vi "Get Tunnel Position on Structure.vi"(8 "error in":errorcluster, 11 "Tunnel Ref":refnum<vi>) -> (0 "error out":errorcluster, 1 "Class Name":string, 2 "Position":cluster{"Left":i32, "Top":i32}, 3 "Tunnel Position":enum16{"Left", "Top", "Right", "Bottom"}(ring))   [LabVIEW 2023]
uses:
  <userlib>/_OpenG.lib/array/array.llb/openg_array.lvlib
panel:
  out "Structure Bounds":T1
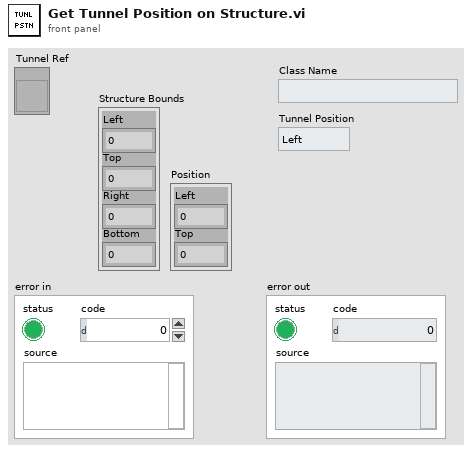
[diagram p1: front panel]
types:
  T1 = cluster{"Left":i16, "Top":i16, "Right":i16, "Bottom":i16}
  T2 = typedef "LVRectTypeDef.ctl" = cluster{"Left":i16, "Top":i16, "Right":i16, "Bottom":i16}
  T3 = typedef "LVPositionTypeDef.ctl" = cluster{"Left":i32, "Top":i32}
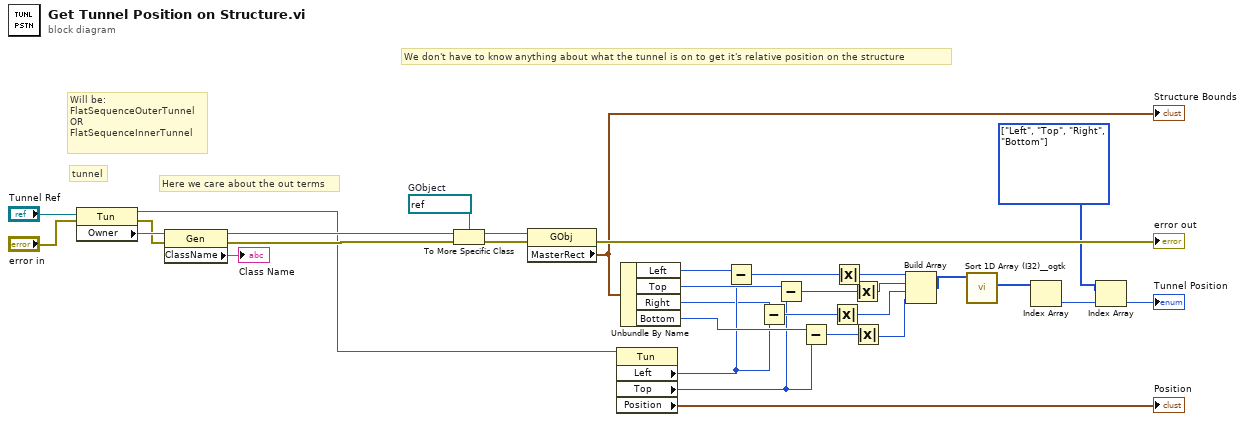
[diagram p0: block diagram]
diagram:
  w19 = enum16{"Left", "Top", "Right", "Bottom"}[] [enum."Left", enum."Top", enum."Right", enum."Bottom"] items=["Left", "Top", "Right", "Bottom"]
  w2 = refnum<vi> refnum  # GObject
  # "We don't have to know anything about what the tunnel is on to get it's relative position on the structure"
  # "Here we care about the out terms"
  # "Will be:\nFlatSequenceOuterTunnel\nOR\nFlatSequenceInnerTunnel"
  # "tunnel"
  n1 = property class="Tun"(reference="Tunnel Ref", error in="error in") -> (reference out=w23:refnum<vi>, error out=w28:errorcluster, "Owner"=w31:refnum<vi>)
  n2 = property class="Gen"(reference=w31, error in=w28) -> (error out=w27:errorcluster, "ClassName"=→"Class Name":string)  [unwired: 1 out]
  n3 = To More Specific Class(target class=w2, reference=w31, error in=w27) -> (specific class reference=w3:refnum<vi>, error out=w1:errorcluster)
  n4 = property class="GObj"(reference=w3, error in=w1) -> (error out=→"error out":errorcluster, "MasterRect"=w22:T2)  [unwired: 1 out]
  "Structure Bounds" <- w22
  n5 = property class="Tun"(reference=w23) -> ("Left"=w6:i32, "Top"=w8:i32, "Position"=→"Position":T3)  [unwired: 1 in, 2 out]
  n6 = Unbundle By Name(w22) -> ("Left"=w4:i16, "Top"=w7:i16, "Right"=w5:i16, "Bottom"=w9:i16)
  n7 = Subtract(x=w4, y=w6) -> (x-y=w10:i32)
  n8 = Subtract(x=w5, y=w6) -> (x-y=w12:i32)
  n9 = Subtract(x=w7, y=w8) -> (x-y=w11:i32)
  n10 = Subtract(x=w9, y=w8) -> (x-y=w13:i32)
  n11 = Absolute Value(x=w12) -> (abs(x)=w16:i32)
  n12 = Absolute Value(x=w10) -> (abs(x)=w14:i32)
  n13 = Absolute Value(x=w11) -> (abs(x)=w15:i32)
  n14 = Absolute Value(x=w13) -> (abs(x)=w17:i32)
  n15 = Build Array(w14, w15, w16, w17) -> (w18:i32[])
  n16 = call <userlib>:"Sort 1D Array (I32)__ogtk.vi"("Array in"=w18) -> ("Sorted Pointers"=w20:i32[])  [unwired: 9 in, 1 out]
  n17 = Index Array(array=w20) -> (element=w21:i32)  [unwired: 1 in]
  n18 = Index Array(array=w19, index=w21) -> (element=→"Tunnel Position":enum16{"Left", "Top", "Right", "Bottom"})
